vi "daqio_replace_dashboard.vi"(8 "error in":errorcluster, 10 "new dashboard string":string, 11 "daq.io type in":T1={"daq.io ref"=refnum, "daq.io API Base"="http://dashboard.daq.io/api/v1", "Device Key"="", "Account ID"="", "online"=TRUE, "SSL"=TRUE, "buffer"=TRUE}) -> (0 "error out":errorcluster, 2 "Dashboard URL":string, 3 "daq.io type out":T1={"daq.io ref"=refnum, "daq.io API Base"="http://dashboard.daq.io/api/v1", "Device Key"="", "Account ID"="", "online"=TRUE, "SSL"=TRUE, "buffer"=TRUE}, 5 "JSON string":string)   [LabVIEW 2013, in "daqio minimal.lvlib"]
doc: "This VI creates a new default dashboard for a specific account and makes it the new default dashboard for the current device."
uses:
  daqio minimal.lvlib
  _typedefs/daqio-Type.ctl
  <vilib>/httpClient/ClientHandle.ctl
  _typedefs/daqio-Device-Just-Dashboards.ctl
  _typedefs/daqio-Device-Dashboards.ctl
  _typedefs/daqio-Device-Put-Dashboards.ctl
  <vilib>/Easy HTTP Client/Easy HTTP.lvlib
  <vilib>/httpClient/LabVIEWHTTPClient.lvlib
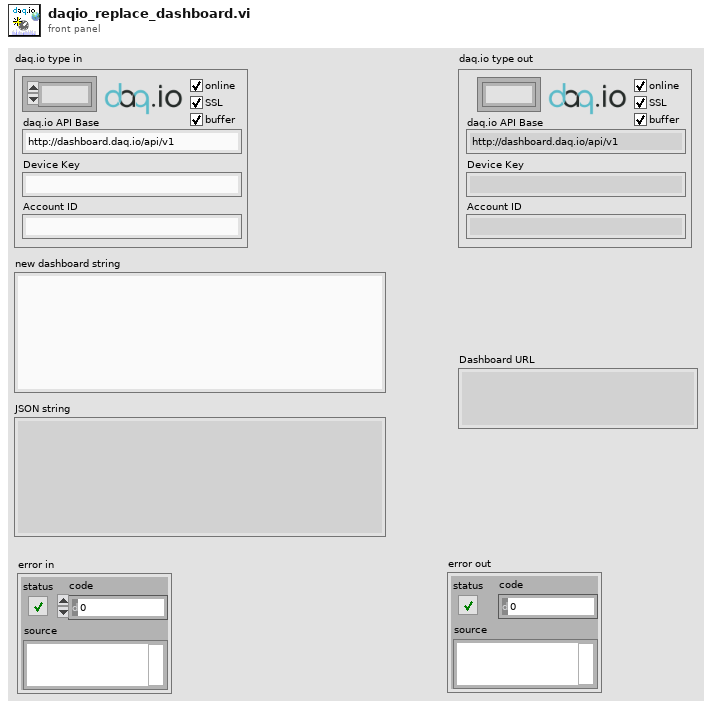
[diagram p1: front panel]
types:
  T1 = typedef "daqio minimal.lvlib/daqio-Type.ctl" = cluster{"daq.io ref":T2, "daq.io API Base":string, "Device Key":string, "Account ID":string, "online":bool, "SSL":bool, "buffer":bool}
  T2 = typedef "LabVIEWHTTPClient.lvlib/ClientHandle.ctl" = refnum<k1>
  T3 = typedef "daqio minimal.lvlib/daqio-Device-Just-Dashboards.ctl" = T4[]
  T4 = typedef "daqio minimal.lvlib/daqio-Device-Dashboards.ctl" = cluster{"active":bool, "definition":string, "_id":string, "label":string}
  T5 = typedef "daqio minimal.lvlib/daqio-Device-Put-Dashboards.ctl" = cluster{"dashboards":T4[]}
  T6 = cluster{"active":bool, "definition":string, "label":string}
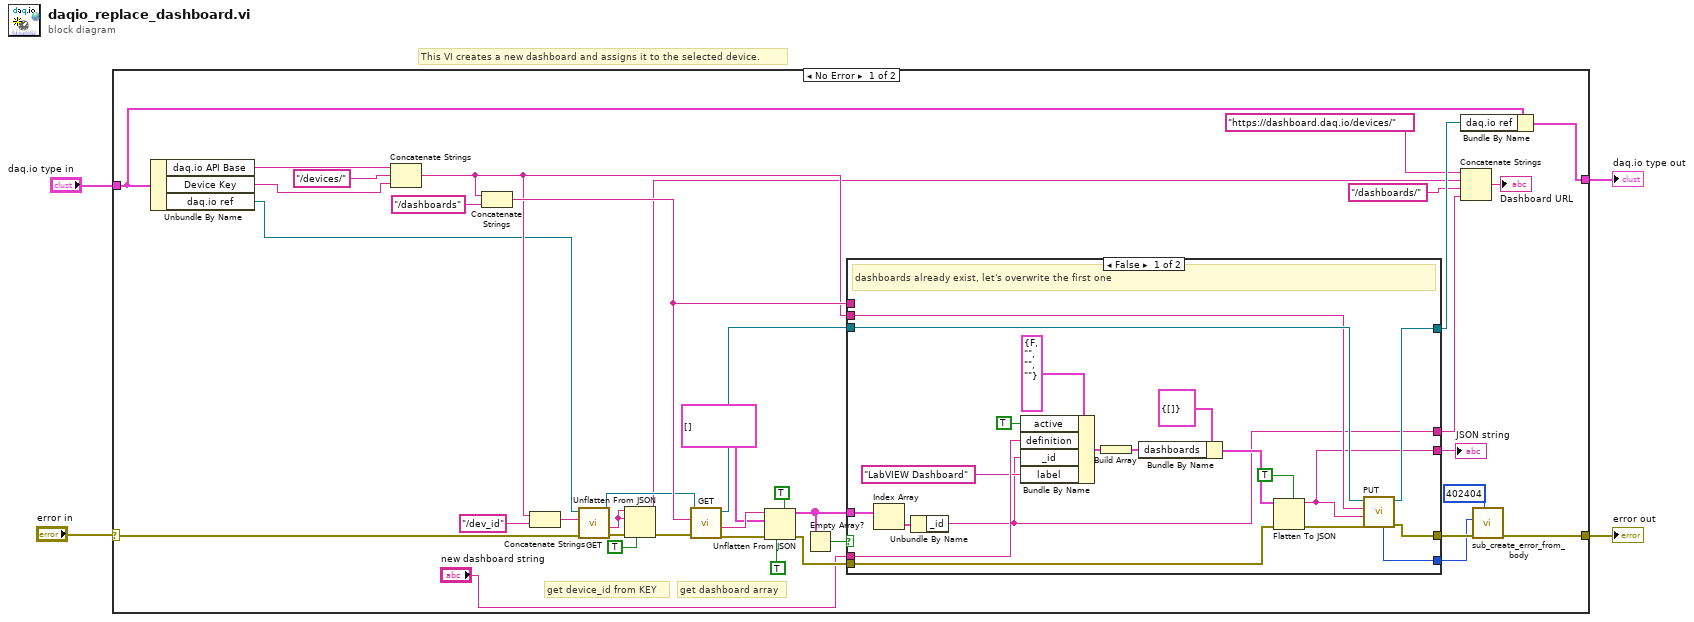
[diagram p0: block diagram]
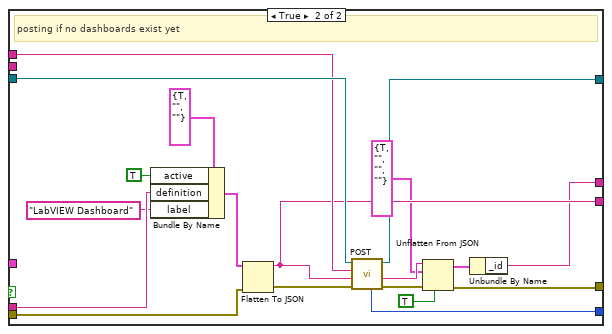
[diagram p2: hidden frame]
diagram:
  # "This VI creates a new dashboard and assigns it to the selected device."
  n1 = case shown="No Error" "error in" {
    selector: "error in" -> [w7 w82]
    tunnel: "daq.io type in" -> [w5 w83]
    tunnel: [w41 w83] -> w3
    tunnel: [w39 w82] -> w2
    frame No Error {
      # "get dashboard array"
      # "get device_id from KEY"
      n2 = Unbundle By Name(w5) -> ("daq.io API Base"=w38:string, "Device Key"=w36:string, "daq.io ref"=w18:T2)
      n3 = Concatenate Strings(w38, "/devices/" ("string"), w36) -> (w20:string)
      n4 = Concatenate Strings(w20, "/dashboards") -> (w24:string)
      n5 = Concatenate Strings(w20, "/dev_id" ("string")) -> (w19:string)
      n6 = call <vilib>:"GET.vi"("error in (no error)"=w7, "url"=w19, "client handle"=w18) -> ("error out"=w9:errorcluster, "body"=w12:string, "client handle out"=w17:T2)  [unwired: 4 in, 2 out]
      n7 = Unflatten From JSON(JSON string=w12, type and defaults=w12, default null elements? (F)=TRUE, error in (no error)=w9) -> (value=w11:string, error out=w8:errorcluster)  [unwired: 3 in]
      n8 = call <vilib>:"GET.vi"("error in (no error)"=w8, "url"=w24, "client handle"=w17) -> ("error out"=w32:errorcluster, "body"=w35:string, "client handle out"=w30:T2)  [unwired: 4 in, 2 out]
      n9 = Unflatten From JSON(enable LabVIEW extensions? (T)=TRUE, JSON string=w35, type and defaults=T3 [] ("dashboards"), default null elements? (F)=TRUE, error in (no error)=w32) -> (value=w26:T3, error out=w31:errorcluster)  [unwired: 2 in]
      n10 = Empty Array?(array=w26) -> (empty?=w13:bool)
      n11 = case shown="False" w13 {
        tunnel: "new dashboard string" -> [w59 w81]
        tunnel: w26 -> [w56 _]
        tunnel: w31 -> [w49 w73]
        tunnel: w30 -> [w55 w79]
        tunnel: w20 -> [w54 _]
        tunnel: [w53 w68] -> w29
        tunnel: [w52 w74] -> w28
        tunnel: [w51 w75] -> w27
        tunnel: [w46 w76] -> w25
        tunnel: w24 -> [_ w78]
        tunnel: [w43 w71] -> w14
        frame False {
          # "dashboards already exist, let's overwrite the first one"
          n12 = Index Array(array=w56) -> (element=w57:T4)  [unwired: 1 in]
          n13 = Unbundle By Name(w57) -> ("_id"=w43:string)
          n14 = Bundle By Name(cluster=T4 {"active"=FALSE, "definition"="", "_id"="", "label"=""} ("dashboard"), "active"=TRUE, "definition"=w59, "_id"=w43, "label"="LabVIEW Dashboard") -> (w60:T4)
          n15 = Build Array(w60) -> (w62:T4[])
          n16 = Bundle By Name(cluster=T5 {"dashboards"=[]} ("Device"), "dashboards"=w62) -> (w50:T5)
          n17 = Flatten To JSON(enable LabVIEW extensions? (T)=TRUE, anything=w50, error in (no error)=w49) -> (JSON string=w46:string, 11:w48:errorcluster)
          n18 = call <vilib>:"PUT.vi"("error in (no error)"=w48, "data"=w46, "url"=w54, "client handle"=w55) -> ("error out"=w53:errorcluster, "client handle out"=w51:T2, "HTTP Response Code"=w52:i32)  [unwired: 3 in, 2 out]
        }
        frame True {
          # "posting if no dashboards exist yet"
          n19 = Bundle By Name(cluster=T6 {"active"=TRUE, "definition"="", "label"=""} ("dashboard"), "active"=TRUE, "definition"=w81, "label"="LabVIEW Dashboard") -> (w72:T6)
          n20 = Flatten To JSON(anything=w72, error in (no error)=w73) -> (JSON string=w76:string, 11:w77:errorcluster)  [unwired: 1 in]
          n21 = call <vilib>:"POST.vi"("error in (no error)"=w77, "data"=w76, "url"=w78, "client handle"=w79) -> ("error out"=w69:errorcluster, "body"=w66:string, "client handle out"=w75:T2, "HTTP Response Code"=w74:i32)  [unwired: 3 in, 1 out]
          n22 = Unflatten From JSON(JSON string=w66, type and defaults=T4 {"active"=TRUE, "definition"="", "_id"="", "label"=""} ("dashboard"), default null elements? (F)=TRUE, error in (no error)=w69) -> (value=w67:T4, error out=w68:errorcluster)  [unwired: 3 in]
          n23 = Unbundle By Name(w67) -> ("_id"=w71:string)
        }
      }
      "JSON string" <- w25
      n24 = Bundle By Name(cluster=w5, "daq.io ref"=w27) -> (w41:T1)
      n25 = Concatenate Strings("https://dashboard.daq.io/devices/" ("string"), w11, "/dashboards/" ("string"), w14) -> (→"Dashboard URL":string)
      n26 = call "sub_create_error_from_body.vi"("error code"=402404, "error in (no error)"=w29, "http code"=w28) -> ("error out"=w39:errorcluster)  [unwired: 8 in]
    }
    frame Error {
    }
  }
  "error out" <- w2
  "daq.io type out" <- w3
